vi "createRational.vi"(1 "real":sgl) -> (0 "rational 2xU32":u32[](array[numeric]))   [LabVIEW 2011]
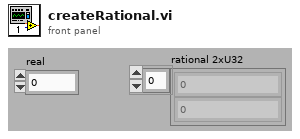
[diagram p1: front panel]
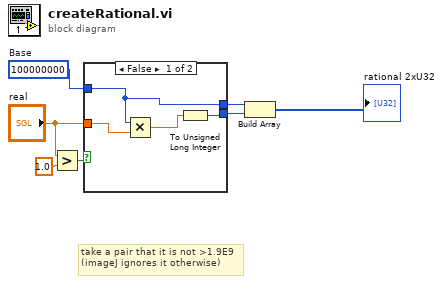
[diagram p0: block diagram]
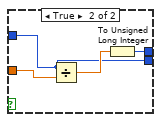
[diagram p2: hidden frame]
diagram:
  w1 = u32 100000000  # Base
  # "take a pair that it is not >1.9E9 \n(imageJ ignores it otherwise)"
  n1 = Greater?(x="real", y=sgl 1.0) -> (0:w3:bool)
  n2 = case shown="False" w3 {
    tunnel: [w9 w12] -> w6
    tunnel: [w8 w15] -> w5
    tunnel: "real" -> [w11 w13]
    tunnel: w1 -> [w8 w12]
    frame False {
      n3 = Multiply(x=w8, y=w11) -> (x*y=w10:sgl)
      n4 = To Unsigned Long Integer(number=w10) -> (unsigned 32bit integer=w9:u32)
    }
    frame True {
      n5 = Divide(x=w12, y=w13) -> (x/y=w14:sgl)
      n6 = To Unsigned Long Integer(number=w14) -> (unsigned 32bit integer=w15:u32)
    }
  }
  n7 = Build Array(w5, w6) -> (→"rational 2xU32":u32[])
